vi "C37 Read BOOL Array from Pointer.vi"(9 "Array Length":i32, 10 "Pointer":u32, 11 "Data is Valid":bool) -> (3 "Values":bool[](array[boolean]))   [LabVIEW 2013, in "C37118-DLL.lvlib"]
uses:
  C37118-DLL.lvlib
  <vilib>/Utility/importsl/GetValueByPointer/GetValueByPointer.xnode
  <vilib>/Utility/importsl/GetValueByPointer/datatype.ctl
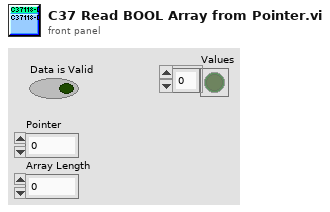
[diagram p1: front panel]
types:
  T1 = enum32{"pack1", "pack2", "pack4", "pack8", "pack16"}
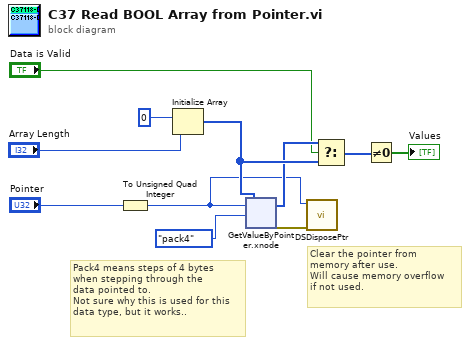
[diagram p0: block diagram]
diagram:
  # "Clear the pointer from \nmemory after use.\nWill cause memory overflow\nif not used."
  # "Pack4 means steps of 4 bytes \nwhen stepping through the \ndata pointed to.\nNot sure why this is used for this\ndata type, but it works.."
  n1 = To Unsigned Quad Integer(1:"Pointer") -> (0:w9:u64)
  n2 = Initialize Array(0 ("digitalValueArr"), "Array Length") -> (w11:i32[])
  n3 = xnode "GetValueByPointer.xnode"("Pointer"=w9, "InputType"=w11, "PackType"=T1."pack4") -> ("Output"=w10:i32[], "ErrorOut"=w8:errorcluster)  [unwired: 1 in]
  n4 = call <vilib>:"DSDisposePtr.vi"("error in (no error)"=w8, "Pointer"=w9) -> ()  [unwired: 9 in, 1 out]
  n5 = Select(t=w10, s="Data is Valid", f=w11) -> (s? t:f=w3:i32[])
  n6 = Not Equal To 0?(x=w3) -> (x != 0?=→"Values":bool[])
